vi "Import.vi"(8 "error in":errorcluster, 11 "Objects in":T1) -> (0 "error out":errorcluster, 1 "Update":bool, 3 "Objects out":T1)   [LabVIEW 2015, in "PID Module editor node.lvclass"]
uses:
  PID Module editor node.lvclass
  <vilib>/NI/DCAF/Tag Editor Core/Table API/Table Manager/object ref.ctl
  <vilib>/NI/DCAF/Tag Editor Core/Configuration Editor/Classes/Engine Parent/Engine Parent Editor Node.lvclass
  <vilib>/NI/DCAF/Tag Editor Core/Configuration Editor/Classes/Module editor node/module editor node.lvclass
  <vilib>/NI/DCAF/Tag Editor Core/Configuration Editor/Classes/Engine Parent/read engine configuration.vi
  <vilib>/NI/DCAF/Tag Editor Core/Configuration Editor/Classes/Engine Parent/write engine configuration.vi
  <vilib>/NI/Module Execution Interface/Engine Configuration/engine configuration.lvclass
  <vilib>/NI/DCAF/Tag Editor Core/Table API/Table Manager/Table Manager.lvclass
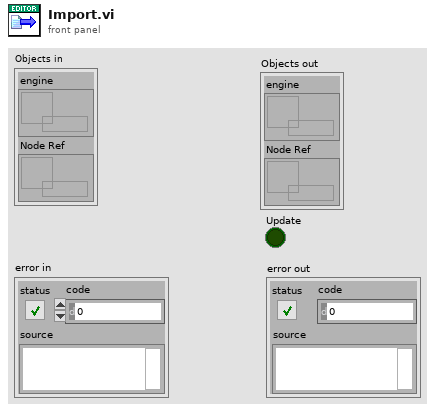
[diagram p1: front panel]
types:
  T1 = typedef "Table Manager.lvlib/Table Manager.lvclass/object ref.ctl" = cluster{"engine":refnum<data-value>, "Node Ref":refnum<data-value>}
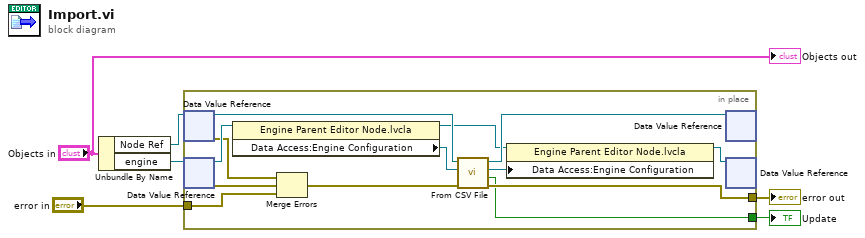
[diagram p0: block diagram]
diagram:
  n1 = Unbundle By Name("Objects in") -> ("Node Ref"=w6:refnum<data-value>, "engine"=w5:refnum<data-value>)
  n2 = in-place {
    in-place-border: "error in" -> [w9]
    in-place-border: [w12] -> w3
    in-place-border: [w7] -> w2
    n3 = in-place-dvr #1(w6) -> (w19:refnum<class "module editor node.lvclass">, w11:errorcluster)
    n4 = in-place-dvr #2(w5) -> (w17:refnum<class "Engine Parent Editor Node.lvclass">, w10:errorcluster)
    n5 = property class="Engine Parent Editor Node.lvcla"(reference=w17) -> (reference out=w14:refnum<class "Engine Parent Editor Node.lvclass">, "Data Access:Engine Configuration"=w16:refnum<class "engine configuration.lvclass">)  [unwired: 1 in, 1 out]
    n6 = Merge Errors(w11, w10, w9) -> (w8:errorcluster)
    n7 = call-dynamic "From CSV File.vi"("error in (no error)"=w8, "engine in"=w16, "module editor node in"=w19) -> ("error out"=w12:errorcluster, "Update"=w7:bool, "engine out"=w15:refnum<class "engine configuration.lvclass">, "module editor node out"=w18:refnum<class "module editor node.lvclass">)  [unwired: 5 in]
    n8 = property class="Engine Parent Editor Node.lvcla"(reference=w14, "Data Access:Engine Configuration"=w15) -> (reference out=w13:refnum<class "Engine Parent Editor Node.lvclass">)  [unwired: 1 in, 1 out]
    n9 = in-place-dvr #1(w18) -> ()  [unwired: 2 out]
    n10 = in-place-dvr #2(w13) -> ()  [unwired: 2 out]
  }
  "error out" <- w3
  "Update" <- w2
  "Objects out" <- "Objects in"
